vi "pmu_Build STAT Field.vi"(11 "measurement data":T1 {"data error" format="%02b"; "PMU time quality" format="%03b"}) -> (3 "STAT field":u16)   [LabVIEW 2013, in "NI_EP_PMU.lvlib"]
uses:
  <vilib>/addons/Electrical Power/PMU/NI_EP_PMU.lvlib
  <vilib>/addons/Electrical Power/PMU/Common/Controls/pmu_Measurement Data (Std 2011).ctl
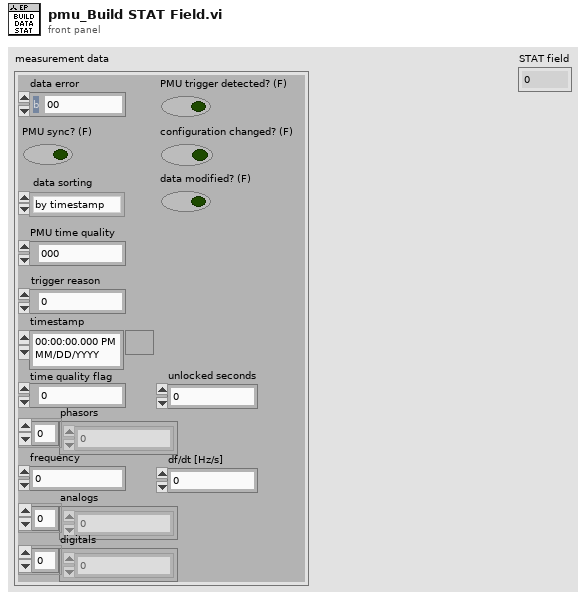
[diagram p1: front panel]
types:
  T1 = typedef "NI_EP_PMU.lvlib/pmu_Measurement Data (Std 2011).ctl" = cluster{"data error":u8, "PMU sync? (F)":bool, "data sorting":enum16{"by timestamp", "by arrival"}, "PMU trigger detected? (F)":bool, "configuration changed? (F)":bool, "data modified? (F)":bool, "PMU time quality":u8, "trigger reason":u8, "timestamp":timestamp, "time quality flag":u8, "unlocked seconds":u32, "phasors":csg[], "frequency":sgl, "df/dt [Hz/s]":sgl, "analogs":sgl[], "digitals":u16[]}
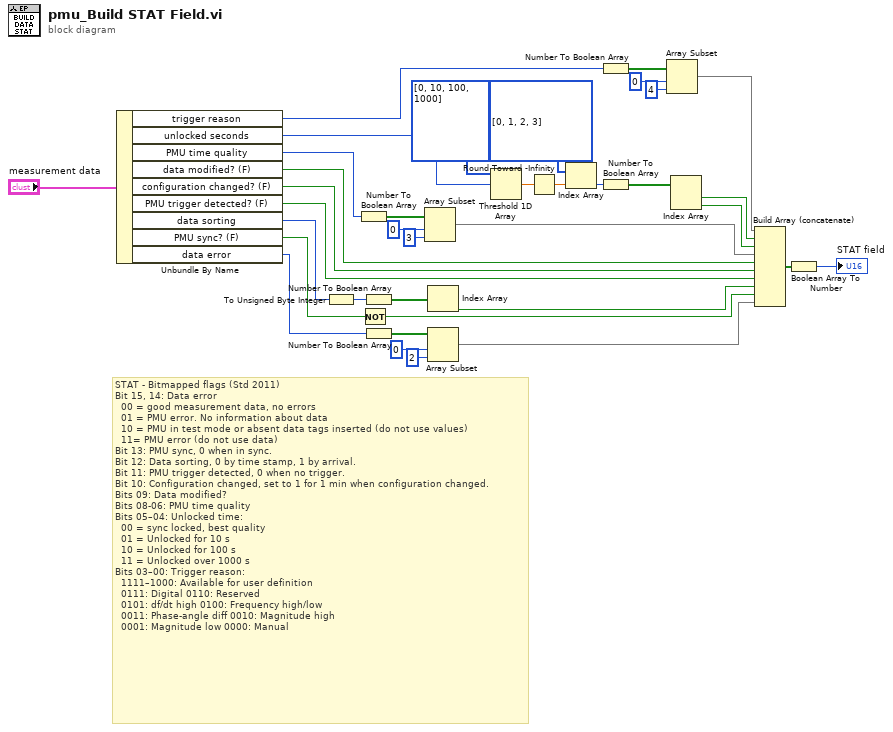
[diagram p0: block diagram]
diagram:
  # "STAT - Bitmapped flags (Std 2011)\nBit 15, 14: Data error\n  00 = good measurement data, no errors\n  01 = PMU error. No information about data\n  10 = PMU in test mode or absent data tags inserted (do not use values)\n  11= PMU error (do not use data)\nBit 13: PMU sync, 0 when in sync.\nBit 12: Data sorting, 0 by time stamp, 1 by arrival.\nBit 11: PMU trigger detected, 0 when no trigger.\nBit 10: Configuration changed, set to 1 for 1 min when configuration changed.\nBits 09: Data modified?\nBits 08-06: PMU time quality\nBits 05–04: Unlocked time:\n  00 = sync locked, best quality\n  01 = Unlocked for 10 s\n  10 = Unlocked for 100 s\n  11 = Unlocked over 1000 s\nBits 03–00: Trigger reason:\n  1111–1000: Available for user definition\n  0111: Digital 0110: Reserved\n  0101: df/dt high 0100: Frequency high/low\n  0011: Phase-angle diff 0010: Magnitude high\n  0001: Magnitude low 0000: Manual"
  n1 = Unbundle By Name("measurement data") -> ("trigger reason"=w9:u8, "unlocked seconds"=w8:u32, "PMU time quality"=w7:u8, "data modified? (F)"=w6:bool, "configuration changed? (F)"=w5:bool, "PMU trigger detected? (F)"=w4:bool, "data sorting"=w3:enum16{"by timestamp", "by arrival"}, "PMU sync? (F)"=w2:bool, "data error"=w1:u8)
  n2 = To Unsigned Byte Integer(number=w3) -> (unsigned 8bit integer=w12:u8)
  n3 = Number To Boolean Array(number=w7) -> (Boolean array=w28:bool[])
  n4 = Not(x=w2) -> (.not. x?=w19:bool)
  n5 = Number To Boolean Array(number=w12) -> (Boolean array=w21:bool[])
  n6 = Number To Boolean Array(number=w1) -> (Boolean array=w15:bool[])
  n7 = Array Subset(array=w28, index=0, length=3) -> (w14:bool[])
  n8 = Index Array(array=w21) -> (element=w20:bool)  [unwired: 1 in]
  n9 = Array Subset(array=w15, index=0, length=2) -> (w13:bool[])
  n10 = Threshold 1D Array(2:w8, 3:u32[] [0, 10, 100, 1000]) -> (0:w36:dbl)  [unwired: 1 in]
  n11 = Round Toward -Infinity(1:w36) -> (0:w35:dbl)
  n12 = Index Array(array=u8[] [0, 1, 2, 3], index=w35) -> (element=w32:u8)
  n13 = Number To Boolean Array(number=w9) -> (Boolean array=w23:bool[])
  n14 = Number To Boolean Array(number=w32) -> (Boolean array=w31:bool[])
  n15 = Array Subset(array=w23, index=0, length=4) -> (w22:bool[])
  n16 = Index Array(array=w31) -> (element #1=w30:bool, element #2=w29:bool)  [unwired: 2 in]
  n17 = Build Array (concatenate)(w22, w30, w29, w14, w6, w5, w4, w20, w19, w13) -> (w18:bool[])
  n18 = Boolean Array To Number(Boolean array=w18) -> (number=→"STAT field":u16)
